vi "Read Laser State.vi"(8 "error in (no error)":errorcluster, 11 "Laser Controller in":refnum<class "Laser Controller.lvclass">) -> (0 "error out":errorcluster, 2 "Laser State":T1, 3 "Laser Controller out":refnum<class "Laser Controller.lvclass">)   [LabVIEW 2022 SP3, in "Laser Controller.lvclass"]
uses:
  Laser Controller.lvclass
  Laser State Data/Laser State.ctl
  Laser Controller.lvclass/Laser Controller.ctl
  Laser State Data/Laser State Data.lvclass/Laser State Data.ctl
  Laser State Data/Laser State Data.lvclass
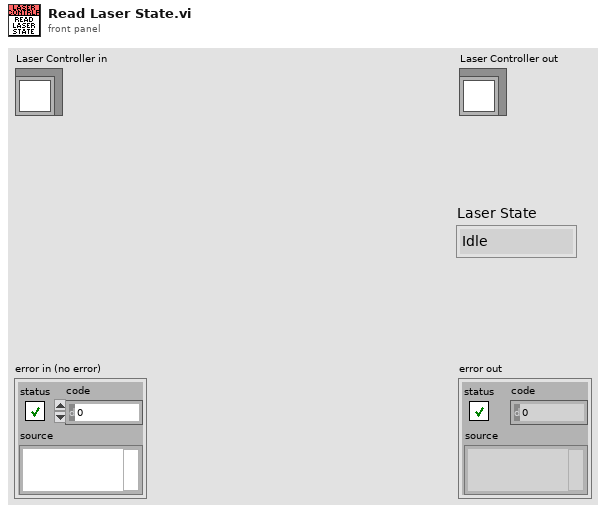
[diagram p1: front panel]
types:
  T1 = typedef "Laser State Data.lvclass/Laser State.ctl" = enum16{"Idle", "Warming", "Ready", "Firing"}
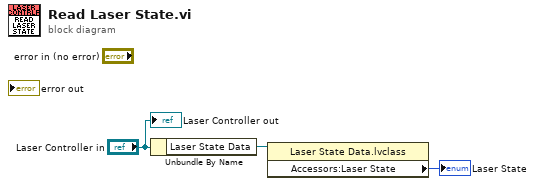
[diagram p0: block diagram]
diagram:
  n1 = Unbundle By Name("Laser Controller in") -> ("Laser State Data"=w2:refnum<data-value>)
  n2 = property class="Laser State Data.lvclass"(reference=w2) -> ("Accessors:Laser State"=→"Laser State":T1)  [unwired: 1 in, 2 out]
  "Laser Controller out" <- "Laser Controller in"
